vi "Data Storage - BRAM FIFO (B256).vi"(0 "data in":T1, 2 "reset":bool, 5 "input valid":bool, 12 "ready for output (T)":bool=TRUE) -> (4 "data out":T1, 6 "output valid":bool, 8 "# of elements to read":u32, 10 "# of elements to write":u32, 14 "ready for input":bool)   [LabVIEW 2018, in "Streaming FPGA.lvlib"]
doc: "BRAM FIFO for elements using the data type provided by the <B>Data Type (B256).ctl</B>. The FIFO implemented by this VI is 512 elements deep.\n\n<B># of elements to read</B> is the number of elements remaining in the FIFO starting from the next cycle.\n<B># of elements to write</B> is the number of empty elements remaining in the FIFO starting from the next cycle."
uses:
  Streaming FPGA.lvlib
  Data Type (B256).ctl
  <vilib>/rvi/DataTransferAndStorage/Container/Common/niFpgaContainerGetUniqueNameForEmu.vi
  <vilib>/rvi/DataTransferAndStorage/Container/Common/niFpgaContainerSetEmuInfo.vi
  <vilib>/rvi/eio/common/nirviEmuReportErrorAndStop.vi
  <vilib>/rvi/DataTransferAndStorage/Container/Common/niFpgaContainerExecOnDevCompGetState.vi
  <vilib>/rvi/Emulation/niFpgaEmulationIsFPGAContextNoSignature.vi
  <vilib>/rvi/Emulation/niFpgaProcessEmulError.vi
  <vilib>/rvi/Emulation/niFpgaSctlEmulationGetInTimedLoop.vi
  <vilib>/rvi/errors/nirviReportUnexpectedCaseInternalError (U32).vi
  <vilib>/rvi/Memory/Memory_Emulation/niFpgaMemoryEmulationCacheClearOnFirstRun.vi
  <vilib>/rvi/Memory/Memory_Emulation/nirvimemoryEmulationManagerCache_MakeExclusive.vi
  <vilib>/rvi/Memory/Memory_Emulation/niFpgaMemoryEmulationValidateCache.vi
  <vilib>/rvi/Memory/Memory_Emulation/nirvimemoryEmulationManagerCache_InsertValue.vi
  <vilib>/Utility/error.llb/Clear Errors.vi
  <vilib>/rvi/Memory/Memory_Emulation/nirvimemoryEmulationManagerCache_ReleaseExclusive.vi
  <vilib>/rvi/Memory/Memory_Emulation/nirvimemoryEmulationManagerCache_GetValue.vi
  <vilib>/rvi/Memory/Memory_Emulation/nirvimemoryEmulationManagerCache_SetValue.vi
  <vilib>/rvi/Emulation/niFpgaSctlEmulationResourceMgr.vi
  <vilib>/rvi/LocalResourceManager/LocalResourceManager.xnode
  <vilib>/rvi/DataTransferAndStorage/Container/XNode/niFpgaContainer.xnode
  <vilib>/rvi/Memory/Memory_Emulation/niFpgaMemoryEmulationRefIn.vi
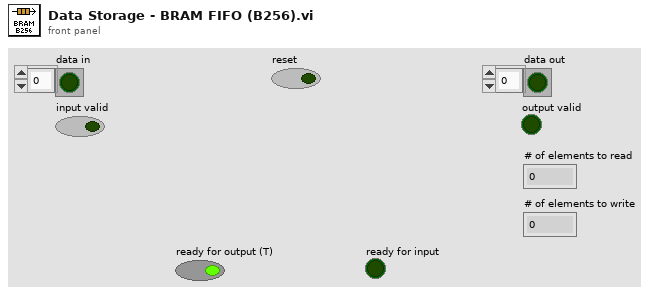
[diagram p1: front panel]
types:
  T1 = typedef "Streaming FPGA.lvlib/Data Type (B256).ctl" = bool[]
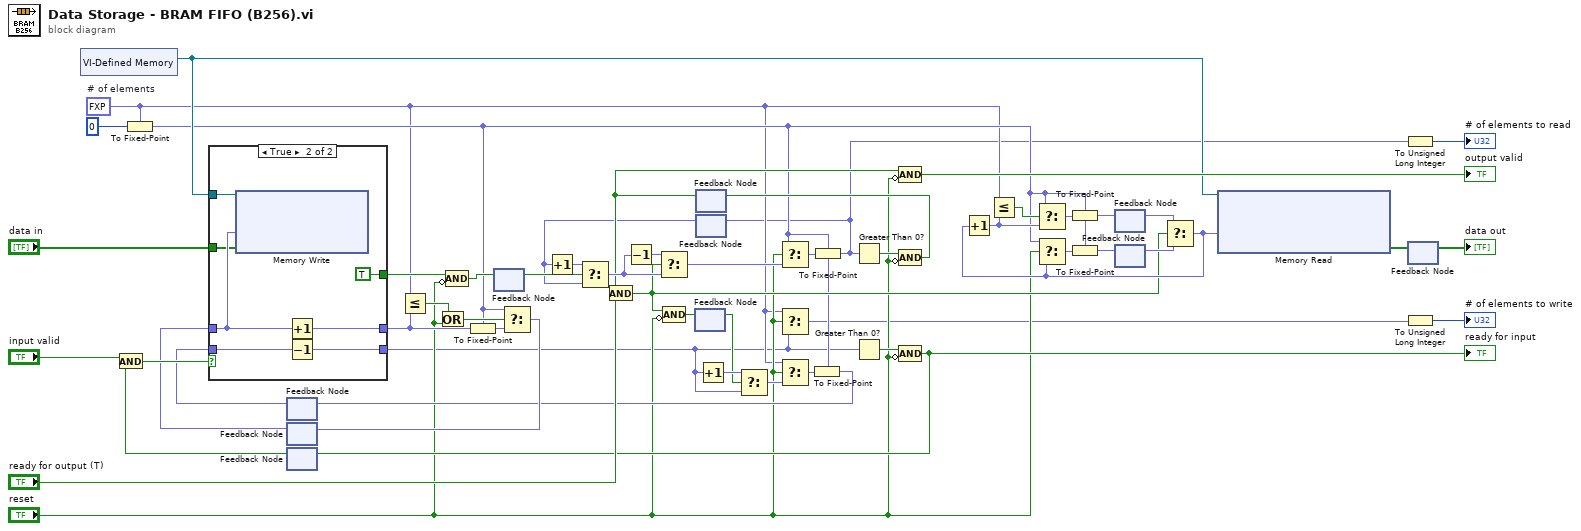
[diagram p0: block diagram]
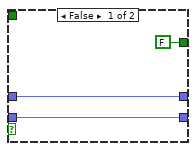
[diagram p2: hidden frame]
diagram:
  w4 = fxp<+,10,10> 512.0  # # of elements
  n1 = xnode "VI-Defined Memory"() -> ("Memory Out"=w48:refnum<k21>)
  n2 = To Fixed-Point(fixed-point type=w4, number=u32 0 ("t")) -> (fixed-point=w8:fxp<+,10,10>)
  n3 = feedback #1() -> (w39:fxp<+,10,10>)  [unwired: 1 in]
  n4 = feedback #2() -> (w37:fxp<+,10,10>)  [unwired: 1 in]
  n5 = feedback #3() -> (w41:bool)  [unwired: 1 in]
  n6 = And(x="input valid", y=w41) -> (x .and. y?=w47:bool)
  n7 = case shown="True" w47 {
    tunnel: w48 -> [_ w65]
    tunnel: w39 -> [w58 w64]
    tunnel: [w58 w63] -> w2
    tunnel: w37 -> [w57 w62]
    tunnel: [w57 w59] -> w18
    tunnel: "data in" -> [_ w61]
    tunnel: [FALSE TRUE] -> w45
    frame False {
    }
    frame True {
      n8 = xnode "Memory Write"("Address"=w62, "Data"=w61, "Memory In"=w65) -> ()  [unwired: 1 out]
      n9 = Increment(x=w62) -> (x+1=w59:fxp<+,11,11>)
      n10 = Decrement(x=w64) -> (x-1=w63:fxp<+/-,11,11>)
    }
  }
  n11 = Less Or Equal?(x=w4, y=w18) -> (x <= y?=w36:bool)
  n12 = Or(x=w36, y="reset") -> (x .or. y?=w35:bool)
  n13 = Compound Arithmetic op=AND(w45, invert "reset") -> (w44:bool)
  n14 = To Fixed-Point(fixed-point type=w8, number=w18) -> (fixed-point=w17:fxp<+,10,10>)
  n15 = feedback #4() -> (w34:bool)  [unwired: 1 in]
  n16 = feedback-in #4(w44) -> ()
  n17 = Select(t=w8, s=w35, f=w17) -> (s? t:f=w38:fxp<+,10,10>)
  n18 = feedback-in #2(w38) -> ()
  n19 = feedback #5() -> (w33:bool)  [unwired: 1 in]
  n20 = feedback #6() -> (w25:bool)  [unwired: 1 in]
  n21 = And(x=w25, y="ready for output (T)") -> (x .and. y?=w24:bool)
  n22 = Compound Arithmetic op=AND(w24, invert "reset") -> (w23:bool)
  n23 = feedback-in #5(w23) -> ()
  n24 = feedback #7() -> (w20:fxp<+,10,10>)  [unwired: 1 in]
  n25 = Increment(x=w20) -> (x+1=w43:fxp<+,11,11>)
  n26 = Select(t=w43, s=w34, f=w20) -> (s? t:f=w31:fxp<+,11,11>)
  n27 = Decrement(x=w31) -> (x-1=w32:fxp<+/-,11,11>)
  n28 = Select(t=w32, s=w24, f=w31) -> (s? t:f=w16:fxp<+/-,12,12>)
  n29 = Increment(x=w2) -> (x+1=w42:fxp<+,11,11>)
  n30 = Select(t=w42, s=w33, f=w2) -> (s? t:f=w40:fxp<+/-,12,12>)
  n31 = Select(t=w8, s="reset", f=w16) -> (s? t:f=w15:fxp<+/-,12,12>)
  n32 = Select(t=w4, s="reset", f=w2) -> (s? t:f=w3:fxp<+/-,11,11>)
  n33 = Select(t=w4, s="reset", f=w40) -> (s? t:f=w14:fxp<+/-,12,12>)
  n34 = To Fixed-Point(fixed-point type=w8, number=w14) -> (fixed-point=w13:fxp<+,10,10>)
  n35 = feedback-in #1(w13) -> ()
  n36 = To Fixed-Point(fixed-point type=w8, number=w15) -> (fixed-point=w1:fxp<+,10,10>)
  n37 = feedback-in #7(w1) -> ()
  n38 = Greater Than 0?(x=w1) -> (x > 0?=w22:bool)
  n39 = Greater Than 0?(x=w2) -> (x > 0?=w46:bool)
  n40 = Compound Arithmetic op=AND(w25, invert "reset") -> (→"output valid":bool)
  n41 = Compound Arithmetic op=AND(w22, invert "reset") -> (w21:bool)
  n42 = feedback-in #6(w21) -> ()
  n43 = Compound Arithmetic op=AND(w46, invert "reset") -> (w51:bool)
  "ready for input" <- w51
  n44 = feedback-in #3(w51) -> ()
  n45 = feedback #8() -> (w30:fxp<+,10,10>)  [unwired: 1 in]
  n46 = feedback #9() -> (w29:fxp<+,10,10>)  [unwired: 1 in]
  n47 = Select(t=w30, s=w24, f=w29) -> (s? t:f=w26:fxp<+,10,10>)
  n48 = Increment(x=w26) -> (x+1=w27:fxp<+,11,11>)
  n49 = Less Or Equal?(x=w4, y=w27) -> (x <= y?=w28:bool)
  n50 = Select(t=w8, s=w28, f=w27) -> (s? t:f=w12:fxp<+,11,11>)
  n51 = Select(t=w8, s="reset", f=w26) -> (s? t:f=w10:fxp<+,10,10>)
  n52 = To Fixed-Point(fixed-point type=w8, number=w12) -> (fixed-point=w11:fxp<+,10,10>)
  n53 = To Fixed-Point(fixed-point type=w8, number=w10) -> (fixed-point=w9:fxp<+,10,10>)
  n54 = feedback-in #8(w11) -> ()
  n55 = feedback-in #9(w9) -> ()
  n56 = xnode "Memory Read"("Address"=w26, "Memory In"=w48) -> ("Data"=w49:bool[])  [unwired: 1 out]
  n57 = To Unsigned Long Integer(number=w1) -> (unsigned 32bit integer=→"# of elements to read":u32)
  n58 = To Unsigned Long Integer(number=w3) -> (unsigned 32bit integer=→"# of elements to write":u32)
  n59 = feedback #10() -> (→"data out":bool[])  [unwired: 1 in]
  n60 = feedback-in #10(w49) -> ()
